vi "LVClass_CameraSet Read AllCameraParametersValue.vi"(8 "error in (no error)":errorcluster, 11 "CameraSet in":refnum<class "CameraSet.lvclass">) -> (0 "error out":errorcluster, 2 "AllCameraParametersValue":T1[](array[typedef]), 3 "CameraSet out":refnum<class "CameraSet.lvclass">)   [LabVIEW 2020, in "CameraSet.lvclass"]
uses:
  CameraSet.lvclass
  CameraParametersSetup.ctl
  CameraParameters_Type.ctl
  CameraSet.lvclass/CameraSet.ctl
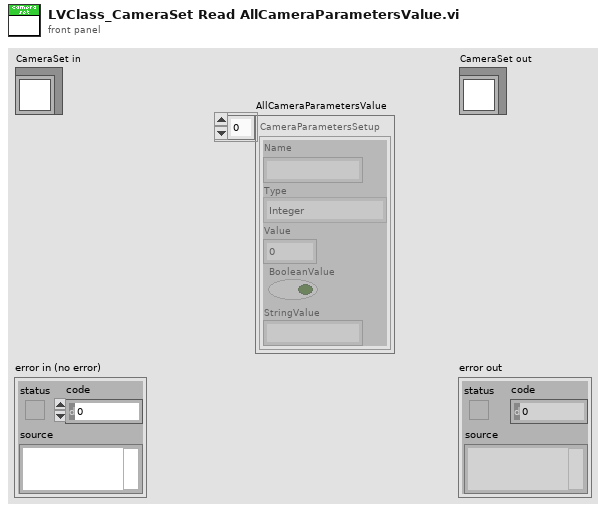
[diagram p1: front panel]
types:
  T1 = typedef "CameraParametersSetup.ctl" = cluster{"Name":string, "Type":T2, "Value":dbl, "BooleanValue":bool, "StringValue":string}
  T2 = typedef "CameraParameters_Type.ctl" = enum16{"Integer", "Real", "String", "Boolean"}
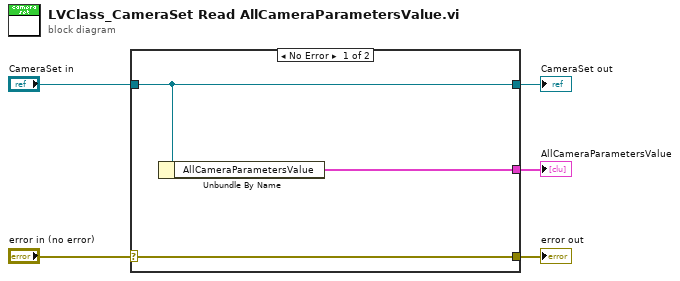
[diagram p0: block diagram]
diagram:
  n1 = case shown="No Error" "error in (no error)" {
    selector: "error in (no error)" -> [w8 w9]
    tunnel: [w8 w9] -> w4
    tunnel: [w7 w10] -> w2
    tunnel: "CameraSet in" -> [w7 w10]
    tunnel: [w6 _] -> w1
    frame No Error {
      n2 = Unbundle By Name(w7) -> ("AllCameraParametersValue"=w6:T1[])
    }
    frame Error {
    }
  }
  "error out" <- w4
  "CameraSet out" <- w2
  "AllCameraParametersValue" <- w1
